vi "main_TMEU.vi"() -> ()   [LabVIEW 2017]
uses:
  <vilib>/Platform/TimedLoop/XDataNode/timing_clust.ctl
  <vilib>/Platform/TimedLoop/XDataNode/nitl_modes.ctl
  <vilib>/Platform/TimedLoop/XDataNode/wakeup.ctl
  <vilib>/platform/TimedLoop/XDataNode/XDataNode.xnode
  <vilib>/Platform/TimedLoop/XDataNode/XDNodeRunTimeDep.lvlib
panel:
  out "dt (sec)":dbl
  out "T3max":dbl
  out "T2max":dbl
  out "T1max":dbl
  out "Boolean 3":bool
  out "Boolean 2":bool
  out "Boolean":bool
  in  "Tab Control":enum32{"Page 1", "Page 2"}(tab)
  out "Sensor3 3":dbl caption="Sensor3"
  out "Sensor2 3":dbl caption="Sensor2"
  out "Sensor1 3":dbl caption="Sensor1"
  out "Sensor3 2":dbl caption="Sensor3"
  out "Sensor2 2":dbl caption="Sensor2"
  out "Sensor1 2":dbl caption="Sensor1"
  out "Sensor3":dbl
  out "Sensor2":dbl
  out "Sensor1":dbl
  out "T3":dbl format="%#.1f"
  out "T2":dbl format="%#.1f"
  out "T1":dbl format="%#.1f"
  out "NI1":tag caption="NI device"
  in  "Exit":bool
  in  "Reset Chart":bool
  in  "Pause Button":bool
  in  "Save as Excel":bool
  in  "Save as image":bool
  out "Temperature Response":cluster{dbl[], dbl[]}[](graph)
  out "dt (ms)":u32
  out "t (sec)":dbl
  in  "tmax":dbl=1.0
  # "Sensors readings"
  # "Temperature Measurements Unit"
  # "Time \nConstant"
  # "Time \nResponse"
  # "Temp.\n@ tau"
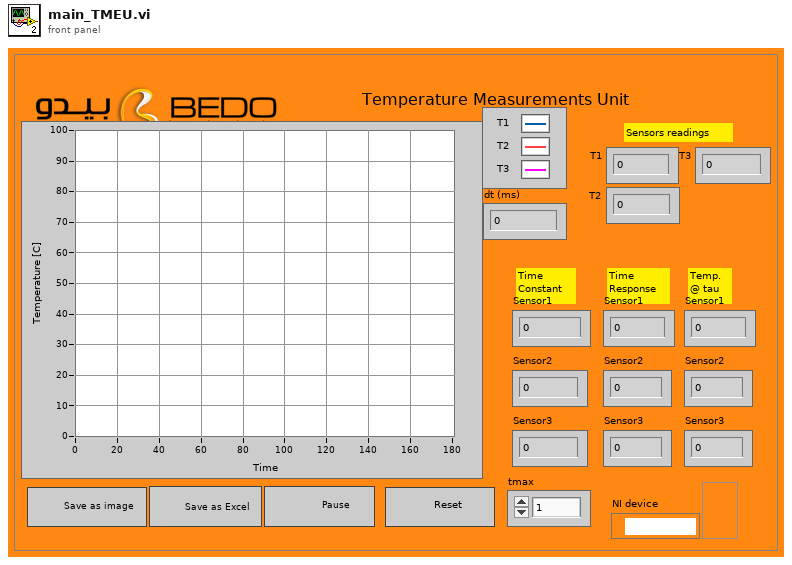
[diagram p1: front panel]
types:
  T1 = enum8{"Enabled", "Disabled", "Disabled and Grayed Out"}
  T2 = typedef "XDNodeRunTimeDep.lvlib/timing_clust.ctl" = cluster{"Expected End [f-1]":u64, "Actual End [f-1]":u64, "Finished Late? [f-1]":bool, "Expected End [i-1]":u64, "Actual End [i-1]":u64, "Finished Late? [i-1]":bool, "Expected Start [i]":u64, "Actual Start [i]":u64, "Expected Start [f]":u64, "Actual Start [f]":u64, "Source Name":string, "Structure Name":string, "Period":i64, "Deadline":i64, "Offset":i64, "Start":i64, "Priority":i32, "Timeout":i32, "Mode":T3, "Wakeup Reason":T4, "Error":errorcluster, "Source Type":string, "Secondary Source Type":string, "Global End Time":u64, "Global Start Time":u64, "Frame Duration":u64, "Iteration Duration":u64, "Assigned CPU":i32, "I/O Scan Engine Mode":u32}
  T3 = typedef "XDNodeRunTimeDep.lvlib/nitl_modes.ctl" = enum32{"No Change", "Process missed periods, maintain original phase", "Discard missed periods, maintain original phase", "Process missed periods, ignore original phase", "Discard missed periods, ignore original phase"}
  T4 = typedef "XDNodeRunTimeDep.lvlib/wakeup.ctl" = enum32{"Normal", "Aborted", "Asynchronous wakeup", "Timing source error", "Timed loop error", "Timeout"}
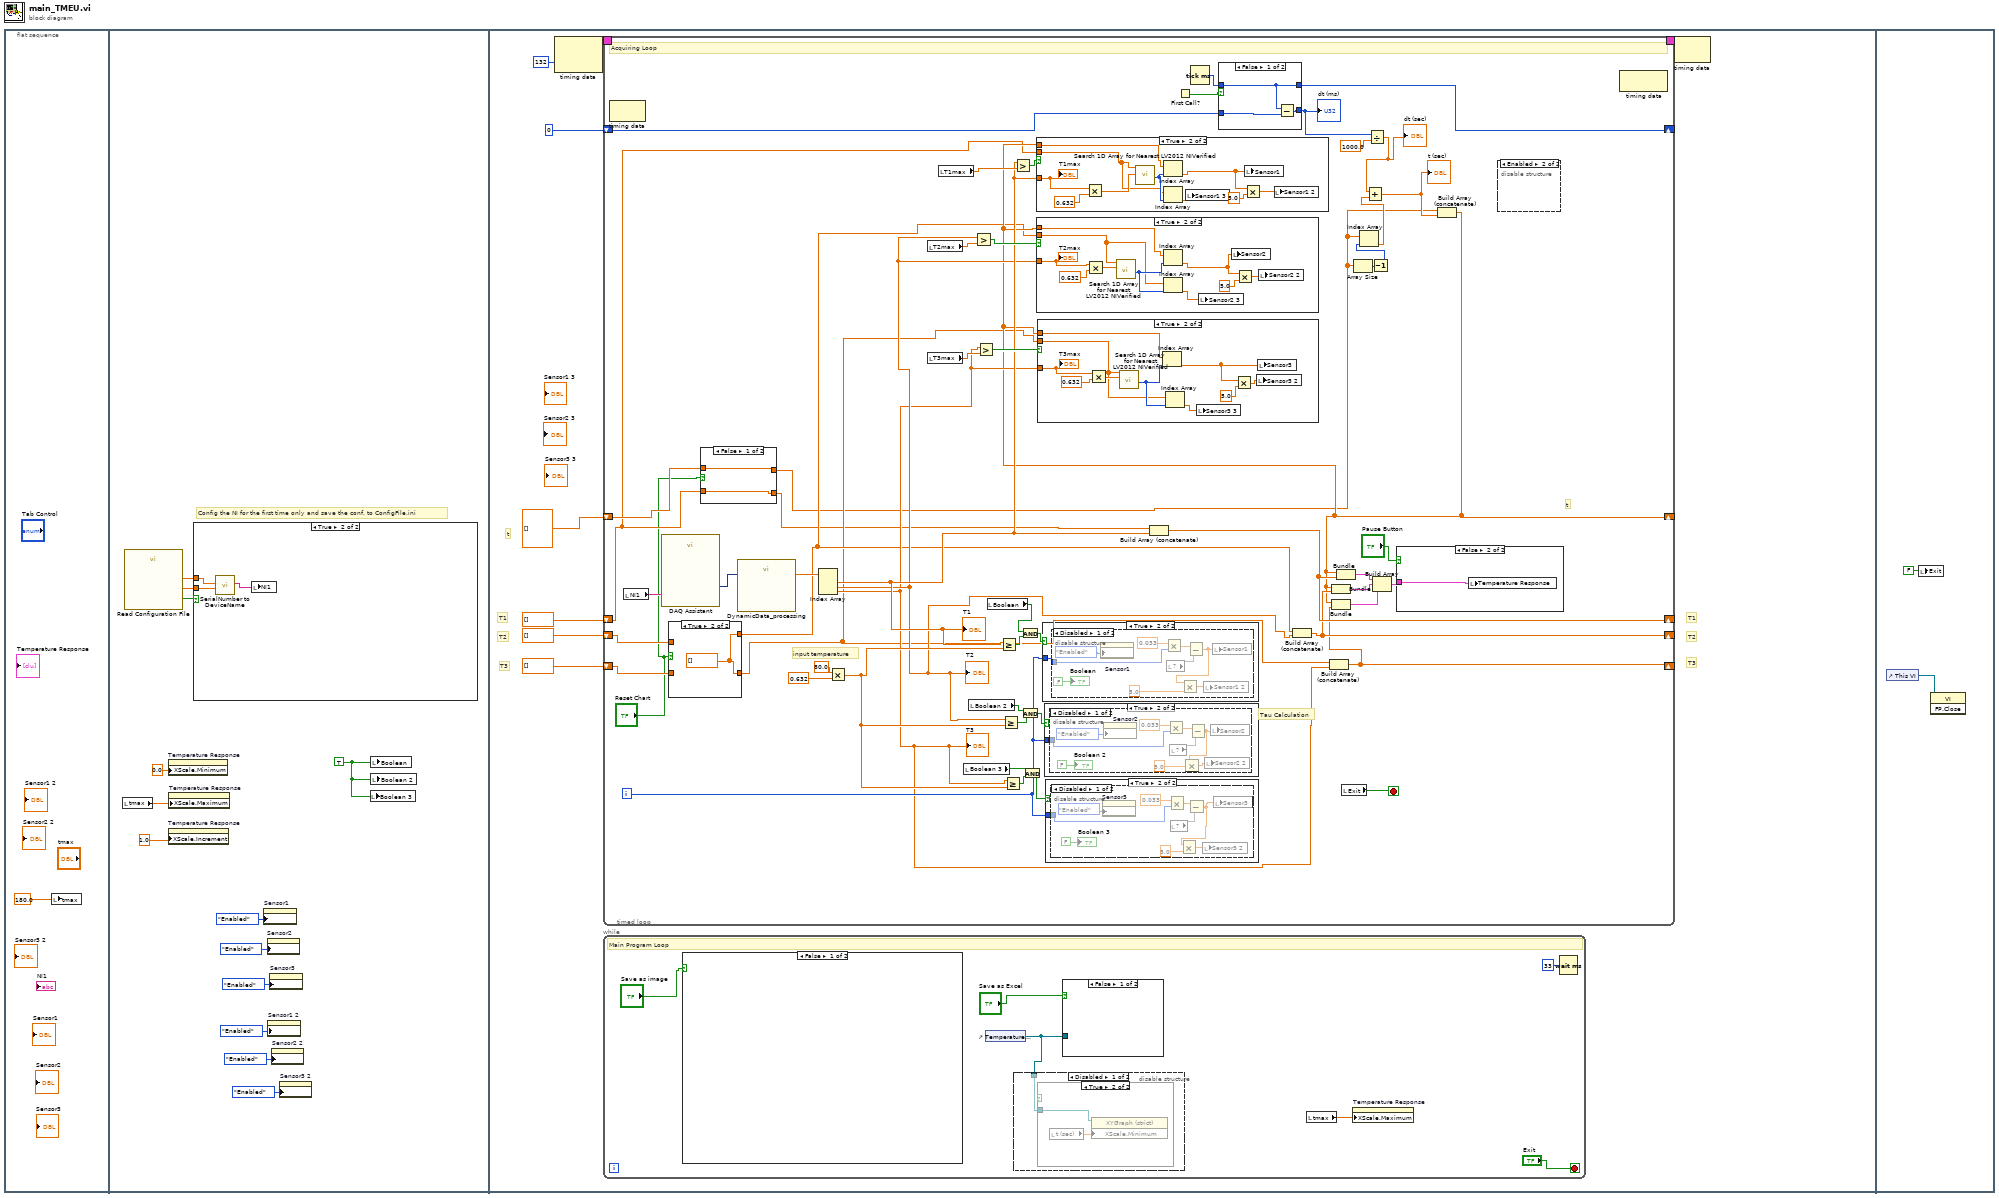
[diagram p0: block diagram]
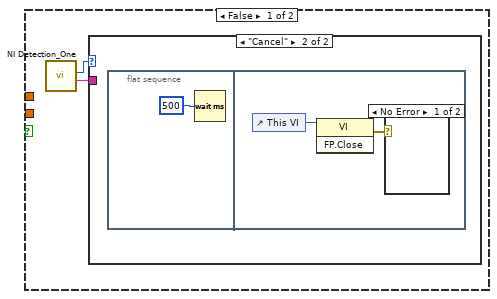
[diagram p2: hidden frame]
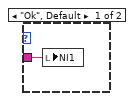
[diagram p3: hidden frame]
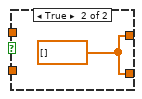
[diagram p5: hidden frame]
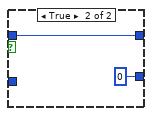
[diagram p7: hidden frame]
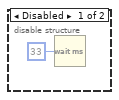
[diagram p8: hidden frame]
diagram:
  n1 = flat-sequence {
    frame #0 {
      n2 = local write "tmax"(180.0 ("tmax")) -> ()
    }
    frame #1 {
      w8 = TRUE ("Boolean")
      # "Config the NI for the first time only and save the conf. to ConfigFile.ini"
      n3 = local read "tmax"() -> (w2:dbl)
      n4 = call "Read Configuration File.vi"() -> ("Serial Numbers Found"=w14:bool, "NI1"=w13:dbl, "NI2"=w12:dbl)  [unwired: 13 in]
      n5 = property on="Temperature Response" class="XYGraph (strict)"("XScale.Minimum"=0.0 ("X Scale.Range:Minimum")) -> ()  [unwired: 2 in, 2 out]
      n6 = property on="Temperature Response" class="XYGraph (strict)"("XScale.Increment"=1.0 ("X Scale.Range:Increment")) -> ()  [unwired: 2 in, 2 out]
      n7 = property on="Temperature Response" class="XYGraph (strict)"("XScale.Maximum"=w2) -> ()  [unwired: 2 in, 2 out]
      n8 = case shown="True" w14 {
        tunnel: w13 -> [_ w23]
        tunnel: w12 -> [_ w22]
        frame False {
          n9 = call "NI Detection_One.vi"() -> ("NI 1"=w15:tag, "Ok/Cancel"=w16:enum16{"Ok", "Cancel"})  [unwired: 8 in, 1 out]
          n10 = case shown="\"Cancel\"" w16 {
            tunnel: w15 -> [w17 _]
            frame "Ok", Default {
              n11 = local write "NI1"(w17) -> ()
            }
            frame "Cancel" {
              n12 = flat-sequence {
                frame #0 {
                  n13 = Wait (ms)(milliseconds to wait=u32 500) -> ()  [unwired: 1 out]
                }
                frame #1 {
                  n14 = control-ref of="This VI"() -> (w20:refnum<vi>)
                  n15 = invoke class="VI" method="FP.Close"(reference=w20) -> (error out=w19:errorcluster)  [unwired: 2 in, 2 out]
                  n16 = case shown="No Error" w19 {
                    frame No Error {
                    }
                    frame Error {
                    }
                  }
                }
              }
            }
          }
        }
        frame True {
          n17 = call "SerialNumber to DeviceName.vi"("NI2 Serial Number"=w22, "NI1 Serial Number"=w23) -> ("NI1 Device Name"=w21:tag)  [unwired: 8 in, 1 out]
          n18 = local write "NI1"(w21) -> ()
        }
      }
      n19 = property on="Sensor1" class="DigNum (strict)"("DisabledEnum"=T1."Enabled" ("Disabled")) -> ()  [unwired: 2 in, 2 out]
      n20 = property on="Sensor2" class="DigNum (strict)"("DisabledEnum"=T1."Enabled" ("Disabled")) -> ()  [unwired: 2 in, 2 out]
      n21 = property on="Sensor1 2" class="DigNum (strict)"("DisabledEnum"=T1."Enabled" ("Disabled")) -> ()  [unwired: 2 in, 2 out]
      n22 = property on="Sensor3" class="DigNum (strict)"("DisabledEnum"=T1."Enabled" ("Disabled")) -> ()  [unwired: 2 in, 2 out]
      n23 = property on="Sensor2 2" class="DigNum (strict)"("DisabledEnum"=T1."Enabled" ("Disabled")) -> ()  [unwired: 2 in, 2 out]
      n24 = property on="Sensor3 2" class="DigNum (strict)"("DisabledEnum"=T1."Enabled" ("Disabled")) -> ()  [unwired: 2 in, 2 out]
      n25 = local write "Boolean 3"(w8) -> ()
      n26 = local write "Boolean"(w8) -> ()
      n27 = local write "Boolean 2"(w8) -> ()
    }
    frame #2 {
      # "t"
      # "T3"
      # "T2"
      # "T1"
      # "T3"
      # "T2"
      # "T1"
      n28 = node-c288(i64 132 ("Period")) -> (w28:T2)  [unwired: 1 in]
      n29 = timed-loop {
        shift-right: [w53] -> _
        shift-left: dbl[] [] -> [w35]
        shift-right: [w52] -> _
        shift-left: dbl[] [] -> [w38]
        shift-right: [w51] -> _
        shift-left: dbl[] [] -> [w37]
        timing: w28 -> [_]
        timing-out: [_] -> w27
        shift-right: [w62] -> _
        shift-left: u32 0 ("millisecond timer value") -> [w61]
        shift-right: [w42] -> _
        shift-left: dbl[] [] -> [w36]
        i -> [w78]
        stop <- w83 stop-if-true
        # "t"
        # "Tau Calculation"
        # "input temperature"
        # "Acquiring Loop"
        n30 = node-c288() -> ()  [unwired: 1 in, 1 out]
        n31 = local read "NI1"() -> (w82:tag)
        n32 = call "DAQ Assistant"("device name"=w82) -> ("data"=w86:dynamicdata)  [unwired: 16 in, 2 out]
        n33 = case shown="True" "Reset Chart" {
          tunnel: [w91 w92] -> w40
          tunnel: [w90 w92] -> w39
          tunnel: w38 -> [w91 _]
          tunnel: w37 -> [w90 _]
          frame False {
          }
          frame True {
            w92 = dbl[] []
          }
        }
        n34 = case shown="False" "Reset Chart" {
          tunnel: [w88 w89] -> w34
          tunnel: [w87 w89] -> w33
          tunnel: w36 -> [w88 _]
          tunnel: w35 -> [w87 _]
          frame False {
          }
          frame True {
            w89 = dbl[] []
          }
        }
        n35 = call "DynamicData_processing.vi"("data"=w86) -> ("DATA"=w85:dbl[])
        n36 = Index Array(array=w85) -> (element #1=w58:dbl, element #2=w57:dbl, element #3=w56:dbl)  [unwired: 3 in]
        "T1" <- w58
        "T2" <- w57
        "T3" <- w56
        n37 = Multiply(x=80.0, y=0.632) -> (x*y=w79:dbl)
        n38 = local read "T2max"() -> (w64:dbl)
        n39 = local read "T3max"() -> (w63:dbl)
        n40 = local read "T1max"() -> (w65:dbl)
        n41 = local read "Boolean 3"() -> (w69:bool)
        n42 = local read "Boolean 2"() -> (w70:bool)
        n43 = Greater?(x=w57, y=w64) -> (0:w67:bool)
        n44 = Greater?(x=w56, y=w63) -> (0:w66:bool)
        n45 = local read "Boolean"() -> (w71:bool)
        n46 = Greater Or Equal?(x=w58, y=w79) -> (x >= y?=w77:bool)
        n47 = Greater Or Equal?(x=w57, y=w79) -> (x >= y?=w76:bool)
        n48 = Greater Or Equal?(x=w56, y=w79) -> (x >= y?=w75:bool)
        n49 = Greater?(x=w58, y=w65) -> (0:w68:bool)
        n50 = And(x=w71, y=w77) -> (x .and. y?=w72:bool)
        n51 = And(x=w70, y=w76) -> (x .and. y?=w73:bool)
        n52 = And(x=w69, y=w75) -> (x .and. y?=w74:bool)
        n53 = case shown="True" w72 {
          tunnel: w78 -> [_ w151]
          frame False {
          }
          frame True {
            n54 = disable-structure shown="Disabled" {
              disable-tunnel: w151 -> [w158 _]
              frame Disabled {
                n55 = property on="Sensor1" class="DigNum (strict)"("DisabledEnum"=T1."Enabled" ("Disabled")) -> ()  [unwired: 2 in, 2 out]
                n56 = Multiply(x=0.033, y=w158) -> (x*y=w156:dbl)
                n57 = local read item#-1() -> (w155)
                n58 = Subtract(x=w156, y=w155) -> (x-y=w154:dbl)
                n59 = Multiply(x=w154, y=5.0) -> (x*y=w153:dbl)
                n60 = local write "Sensor1 2"(w153) -> ()
                n61 = local write "Sensor1"(w154) -> ()
                "Boolean" <- FALSE
              }
              frame Enabled {
              }
            }
          }
        }
        n62 = case shown="True" w73 {
          tunnel: w78 -> [_ w141]
          frame False {
          }
          frame True {
            n63 = disable-structure shown="Disabled" {
              disable-tunnel: w141 -> [w149 _]
              frame Disabled {
                n64 = property on="Sensor2" class="DigNum (strict)"("DisabledEnum"=T1."Enabled" ("Disabled")) -> ()  [unwired: 2 in, 2 out]
                n65 = Multiply(x=0.033, y=w149) -> (x*y=w147:dbl)
                n66 = local read item#-1() -> (w146)
                n67 = Subtract(x=w147, y=w146) -> (x-y=w145:dbl)
                n68 = Multiply(x=w145, y=5.0) -> (x*y=w143:dbl)
                n69 = local write "Sensor2 2"(w143) -> ()
                n70 = local write "Sensor2"(w145) -> ()
                "Boolean 2" <- FALSE
              }
              frame Enabled {
              }
            }
          }
        }
        n71 = case shown="True" w74 {
          tunnel: w78 -> [_ w131]
          frame False {
          }
          frame True {
            n72 = disable-structure shown="Disabled" {
              disable-tunnel: w131 -> [w139 _]
              frame Disabled {
                n73 = property on="Sensor3" class="DigNum (strict)"("DisabledEnum"=T1."Enabled" ("Disabled")) -> ()  [unwired: 2 in, 2 out]
                n74 = Multiply(x=0.033, y=w139) -> (x*y=w137:dbl)
                n75 = local read item#-1() -> (w136)
                n76 = Subtract(x=w137, y=w136) -> (x-y=w133:dbl)
                n77 = Multiply(x=w133, y=5.0) -> (x*y=w135:dbl)
                n78 = local write "Sensor3 2"(w135) -> ()
                n79 = local write "Sensor3"(w133) -> ()
                "Boolean 3" <- FALSE
              }
              frame Enabled {
              }
            }
          }
        }
        n80 = Build Array (concatenate)(w33, w58) -> (w53:dbl[])
        n81 = First Call?() -> (First Call?: T/F=w46:bool)
        n82 = Tick Count (ms)() -> (millisecond timer value=w45:u32)
        n83 = case shown="False" w46 {
          tunnel: [w93 w97] -> w62
          tunnel: w61 -> [w95 _]
          tunnel: [w94 u32 0] -> w60
          tunnel: w45 -> [w93 w97]
          frame False {
            n84 = Subtract(x=w93, y=w95) -> (x-y=w94:u32)
          }
          frame True {
          }
        }
        "dt (ms)" <- w60
        n85 = Build Array (concatenate)(w40, w57) -> (w52:dbl[])
        n86 = Build Array (concatenate)(w39, w56) -> (w51:dbl[])
        n87 = local read "Exit"() -> (w83:bool)
        n88 = Array Size(array=w34) -> (size(s)=w44:i32)
        n89 = Divide(x=w60, y=1000.0) -> (x/y=w55:dbl)
        "dt (sec)" <- w55
        n90 = Decrement(x=w44) -> (x-1=w43:i32)
        n91 = Index Array(array=w34, index=w43) -> (element=w54:dbl)
        n92 = Add(x=w55, y=w54) -> (x+y=w41:dbl)
        "t (sec)" <- w41
        n93 = Build Array (concatenate)(w34, w41) -> (w42:dbl[])
        n94 = case shown="True" w68 {
          tunnel: w58 -> [_ w129]
          tunnel: w35 -> [_ w122]
          tunnel: w42 -> [_ w125]
          frame False {
          }
          frame True {
            n95 = Multiply(x=w129, y=0.632) -> (x*y=w126:dbl)
            n96 = call "Search 1D Array for Nearest LV2012 NIVerified.vi"("desired element"=w126, "1D Array"=w122) -> ("closest index"=w123:i32)  [unwired: 8 in, 1 out]
            n97 = Index Array(array=w125, index=w123) -> (element=w124:dbl)
            n98 = Index Array(array=w122, index=w123) -> (element=w121:dbl)
            n99 = local write "Sensor1 3"(w121) -> ()
            n100 = Multiply(x=w124, y=5.0) -> (x*y=w127:dbl)
            n101 = local write "Sensor1"(w124) -> ()
            n102 = local write "Sensor1 2"(w127) -> ()
            "T1max" <- w129
          }
        }
        n103 = case shown="True" w67 {
          tunnel: w57 -> [_ w119]
          tunnel: w40 -> [_ w112]
          tunnel: w42 -> [_ w115]
          frame False {
          }
          frame True {
            n104 = Multiply(x=w119, y=0.632) -> (x*y=w118:dbl)
            n105 = call "Search 1D Array for Nearest LV2012 NIVerified.vi"("desired element"=w118, "1D Array"=w112) -> ("closest index"=w113:i32)  [unwired: 8 in, 1 out]
            n106 = Index Array(array=w115, index=w113) -> (element=w114:dbl)
            n107 = Index Array(array=w112, index=w113) -> (element=w111:dbl)
            n108 = local write "Sensor2 3"(w111) -> ()
            n109 = local write "Sensor2"(w114) -> ()
            n110 = Multiply(x=w114, y=5.0) -> (x*y=w116:dbl)
            n111 = local write "Sensor2 2"(w116) -> ()
            "T2max" <- w119
          }
        }
        n112 = case shown="True" w66 {
          tunnel: w56 -> [_ w110]
          tunnel: w39 -> [_ w102]
          tunnel: w42 -> [_ w105]
          frame False {
          }
          frame True {
            n113 = Multiply(x=w110, y=0.632) -> (x*y=w108:dbl)
            n114 = call "Search 1D Array for Nearest LV2012 NIVerified.vi"("desired element"=w108, "1D Array"=w102) -> ("closest index"=w103:i32)  [unwired: 8 in, 1 out]
            n115 = Index Array(array=w105, index=w103) -> (element=w104:dbl)
            n116 = Index Array(array=w102, index=w103) -> (element=w101:dbl)
            n117 = local write "Sensor3 3"(w101) -> ()
            n118 = Multiply(x=w104, y=5.0) -> (x*y=w106:dbl)
            n119 = local write "Sensor3 2"(w106) -> ()
            n120 = local write "Sensor3"(w104) -> ()
            "T3max" <- w110
          }
        }
        n121 = Bundle(w42, w52) -> (w49:cluster{dbl[], dbl[]})  [unwired: 1 in]
        n122 = Bundle(w42, w51) -> (w48:cluster{dbl[], dbl[]})  [unwired: 1 in]
        n123 = Bundle(w42, w53) -> (w50:cluster{dbl[], dbl[]})  [unwired: 1 in]
        n124 = Build Array(w50, w49, w48) -> (w47:cluster{dbl[], dbl[]}[])
        n125 = case shown="False" "Pause Button" {
          tunnel: w47 -> [_ w161]
          frame True {
          }
          frame False {
            n126 = local write "Temperature Response"(w161) -> ()
          }
        }
        n127 = disable-structure shown="Enabled" {
          frame Disabled {
            n128 = Wait (ms)(milliseconds to wait=u32 33) -> ()  [unwired: 1 out]
          }
          frame Enabled {
          }
        }
        n129 = node-c288() -> ()  [unwired: 1 in, 1 out]
      }
      n130 = while {
        stop <- "Exit" stop-if-true
        # "Main Program Loop"
        n131 = case shown="False" "Save as image" {
          frame False {
          }
          frame True {
            n132 = control-ref of="Temperature Response"() -> (w176:refnum<vi>)
            n133 = call "File Dialog"("prompt"="Save File", "button label"="Save", "pattern (all files)"="*.BMP", "pattern label"="Picture") -> ("selected path"=w178:path, "cancelled"=w177:bool, "error out"=w179:errorcluster)  [unwired: 8 in, 1 out]
            n134 = case shown="Error" w179 {
              frame No Error {
              }
              frame Error {
              }
            }
            n135 = case shown="False" w177 {
              tunnel: w178 -> [w186 _]
              tunnel: w176 -> [w184 _]
              frame False {
                n136 = invoke on="Invoke Node" class="XYGraph (strict)" method="Export Image"(reference=w184, "FileType"=enum32{"BMP", "EPS", "EMF", "PICT"}."BMP" ("File Type"), "Target"=enum32{"File", "Clipboard"}."File", "Path"=w186, "HideGrid"=FALSE ("Hide Grid")) -> ()  [unwired: 3 in, 8 out]
              }
              frame True {
              }
            }
          }
        }
        n137 = control-ref of="Temperature Response"() -> (w168:refnum<vi>)
        n138 = disable-structure shown="Disabled" {
          disable-tunnel: w168 -> [w172 _]
          frame Disabled {
            n139 = case shown="True" {
              selector: _ -> [_ _]
              tunnel: w172 -> [_ w174]
              frame False {
              }
              frame True {
                n140 = local read "t (sec)"() -> (w173:dbl)
                n141 = property on="Property Node" class="XYGraph (strict)"(reference=w174, "XScale.Minimum"=w173) -> ()  [unwired: 1 in, 2 out]
              }
            }
          }
          frame Enabled {
          }
        }
        n142 = case shown="False" "Save as Excel" {
          tunnel: w168 -> [_ w175]
          frame False {
          }
          frame True {
            n143 = invoke on="Invoke Node" class="XYGraph (strict)" method="Export Data to Excel"(reference=w175) -> ()  [unwired: 2 in, 3 out]
          }
        }
        n144 = local read "tmax"() -> (w166:dbl)
        n145 = property on="Temperature Response" class="XYGraph (strict)"("XScale.Maximum"=w166) -> ()  [unwired: 2 in, 2 out]
        n146 = Wait (ms)(milliseconds to wait=u32 33) -> ()  [unwired: 1 out]
      }
      n147 = node-c288(w27) -> ()  [unwired: 1 out]
    }
    frame #3 {
      n148 = control-ref of="This VI"() -> (w189:refnum<vi>)
      n149 = local write "Exit"(FALSE ("Exit")) -> ()
      n150 = invoke class="VI" method="FP.Close"(reference=w189) -> ()  [unwired: 2 in, 3 out]
    }
  }
